vi "Pcre2SubstringCopyByNumber8.vi"(8 "error in":errorcluster, 9 "Length":u64, 10 "Number":i32, 11 "pMatchData":u64 format="%.0x") -> (0 "error out":errorcluster, 2 "Substring":string, 3 "pMatchData":u64 format="%.0x")   [LabVIEW 2021, in "libpcre2-8.lvlib"]
uses:
  libpcre2-8.lvlib
  libpcre2-8-x32.dll
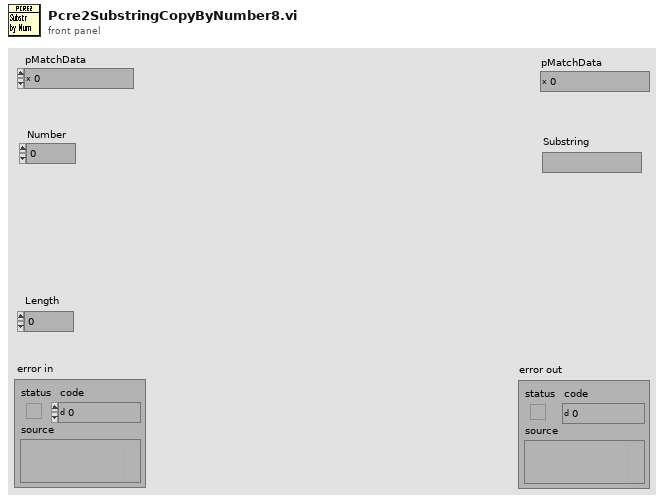
[diagram p1: front panel]
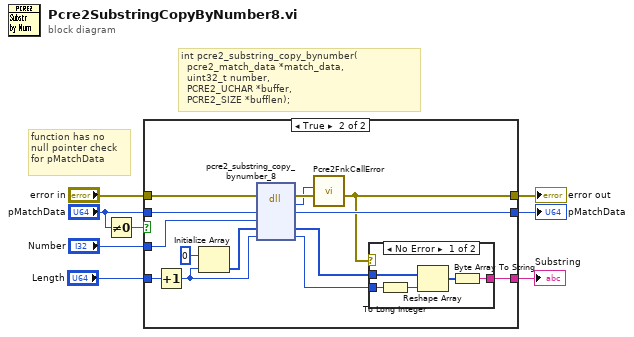
[diagram p0: block diagram]
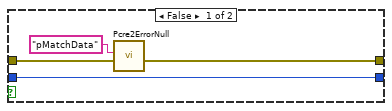
[diagram p2: hidden frame]
diagram:
  # "function has no \nnull pointer check \nfor pMatchData"
  # "int pcre2_substring_copy_bynumber(\n  pcre2_match_data *match_data, \n  uint32_t number, \n  PCRE2_UCHAR *buffer, \n  PCRE2_SIZE *bufflen);"
  n1 = Not Equal To 0?(x="pMatchData") -> (x != 0?=w5:bool)
  n2 = case shown="True" w5 {
    tunnel: "error in" -> [w11 w24]
    tunnel: [w9 w17] -> w7
    tunnel: "pMatchData" -> [w12 w23]
    tunnel: [w12 w22] -> w6
    tunnel: "Number" -> [_ w21]
    tunnel: "Length" -> [_ w20]
    tunnel: [_ w16] -> w2
    frame False {
      n3 = call "Pcre2ErrorNull.vi"("error in"=w11, "What"="pMatchData" ("message")) -> ("error out"=w9:errorcluster)  [unwired: 9 in]
    }
    frame True {
      n4 = Increment(x=w20) -> (x+1=w14:u64)
      n5 = Initialize Array(u8 0 ("U8"), w14) -> (w13:u8[])
      n6 = dll-call lib="libpcre2-8-x*.dll" fn="pcre2_substring_copy_bynumber_8"(error in=w24, "match_data"=w23, "number"=w21, "buffer"=w13, "buflen"=w14) -> (error out=w19:errorcluster, "return type"=w18:i32, "match_data"=w22:u64, "buffer"=w26:u8[], "buflen"=w25:u64)  [unwired: 3 in, 1 out]
      n7 = call "Pcre2FnkCallError.vi"("error in"=w19, "ErrorCode"=w18) -> ("error out"=w17:errorcluster)  [unwired: 9 in]
      n8 = case shown="No Error" w17 {
        tunnel: w26 -> [w31 _]
        tunnel: w25 -> [w29 _]
        tunnel: [w27 _] -> w16
        frame No Error {
          n9 = To Long Integer(number=w29) -> (32bit integer=w28:i32)
          n10 = Reshape Array(w31, w28) -> (w30:u8[])
          n11 = Byte Array To String(unsigned byte array=w30) -> (string=w27:string)
        }
        frame Error {
        }
      }
    }
  }
  "pMatchData" <- w6
  "error out" <- w7
  "Substring" <- w2
